vi "Inpaint.vi"(0 "image in":refnum<class "MSC Image.lvclass">, 1 "mask image in":refnum<class "MSC Image.lvclass">, 2 "Radius":i32=5, 3 "Algorithm":T1, 5 "error in (no error)":errorcluster) -> (14 "image out":refnum<class "MSC Image.lvclass">, 15 "mask image out":refnum<class "MSC Image.lvclass">, 19 "error out":errorcluster)   [LabVIEW 2016, in "MSC Image.lvclass"]
doc: "Restores marked image regions through an inpaint algorithm."
uses:
  MSC Image.lvclass
  Dependencies/x86/MSC I Process32.dll
  controls/Inpaint Algorithm Method.ctl
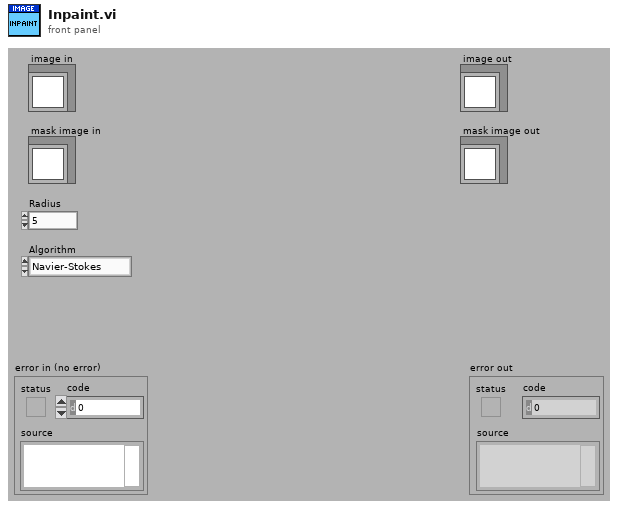
[diagram p1: front panel]
types:
  T1 = typedef "MSC Image.lvclass/Inpaint Algorithm Method.ctl" = enum16{"Navier-Stokes", "Alexandru Telea"}
  T2 = typedef "Image.ctl" = cluster{"Pointer":u64, "Size":T3, "Image Type":T4, "Time Stamp":timestamp, "Variant":variant}
  T3 = typedef "Size.ctl" = cluster{"Cols":i32, "Rows":i32}
  T4 = typedef "Image Type.ctl" = i32
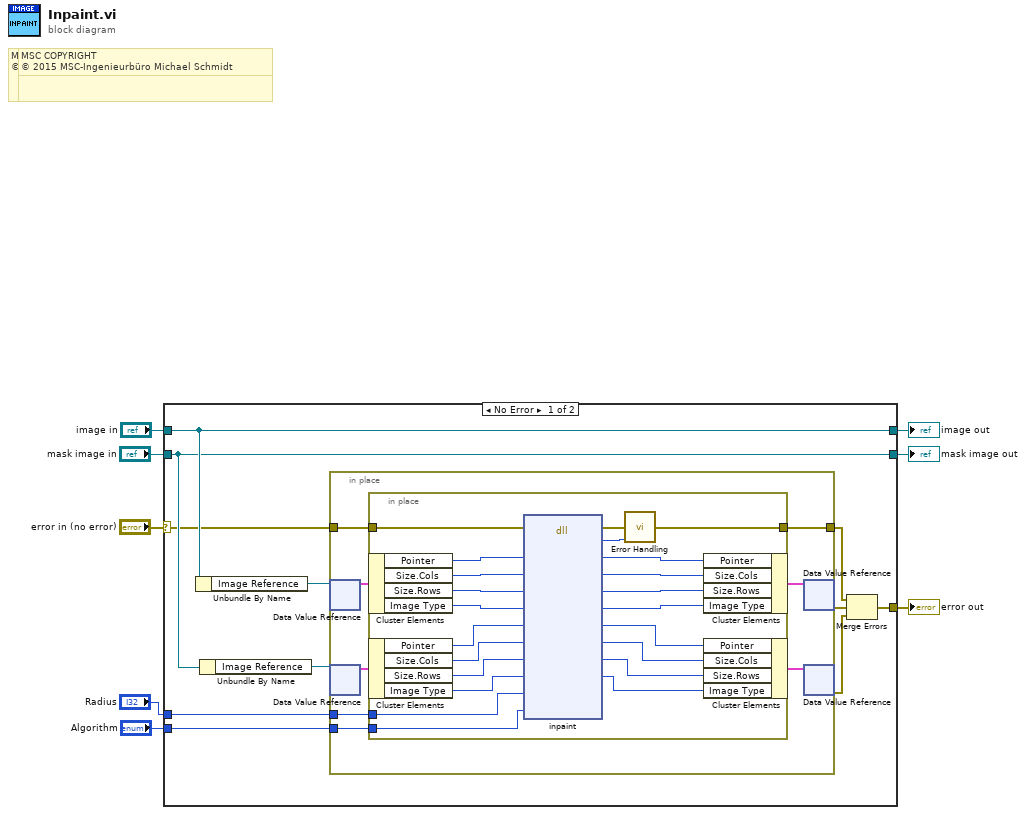
[diagram p0: block diagram]
diagram:
  # "MSC COPYRIGHT\n© 2016 MSC-Ingenieurbüro Michael Schmidt"
  # "MSC COPYRIGHT\n© 2016 MSC-Ingenieurbüro Michael Schmidt"
  # "MSC COPYRIGHT\n© 2015 MSC-Ingenieurbüro Michael Schmidt"
  # "MSC COPYRIGHT\n© 2015 MSC-Ingenieurbüro Michael Schmidt"
  n1 = case shown="No Error" "error in (no error)" {
    selector: "error in (no error)" -> [w9 w52]
    tunnel: [w16 w52] -> w1
    tunnel: [w10 w50] -> w6
    tunnel: "image in" -> [w13 w51]
    tunnel: [w13 w51] -> w7
    tunnel: "mask image in" -> [w10 w50]
    tunnel: "Radius" -> [w15 _]
    tunnel: "Algorithm" -> [w14 _]
    frame No Error {
      n2 = Unbundle By Name(w13) -> ("Image Reference"=w12:refnum<data-value>)
      n3 = Unbundle By Name(w10) -> ("Image Reference"=w11:refnum<data-value>)
      n4 = in-place {
        in-place-border: w9 -> [w25]
        in-place-border: [w24] -> w19
        in-place-border: w15 -> [w21]
        in-place-border: w14 -> [w20]
        n5 = in-place-dvr #1(w12) -> (w26:T2)  [unwired: 1 out]
        n6 = in-place-dvr #2(w11) -> (w23:T2)  [unwired: 1 out]
        n7 = in-place {
          in-place-border: w25 -> [w30]
          in-place-border: [w49] -> w24
          in-place-border: w21 -> [w29]
          in-place-border: w20 -> [w28]
          n8 = in-place-cluster #3(w26) -> ("Pointer"=w48:u64, "Size.Cols"=w47:i32, "Size.Rows"=w46:i32, "Image Type"=w45:T4)
          n9 = in-place-cluster #4(w23) -> ("Pointer"=w44:u64, "Size.Cols"=w43:i32, "Size.Rows"=w42:i32, "Image Type"=w41:T4)
          n10 = dll-call lib="C:/Users/MSC/LabVIEW Projekte/LV 2014/MSC I-Process/user.lib/MSC-I Process/Dependencies/x86/MSC I Process*.dll" fn="inpaint"(error in=w30, "pointer"=w48, "cols"=w47, "rows"=w46, "type"=w45, "pointerMask"=w44, "colsMask"=w43, "rowsMask"=w42, "typeMask"=w41, "radius"=w29, "flag"=w28) -> (error out=w31:errorcluster, "error"=w32:i32, "pointer"=w36:u64, "cols"=w35:i32, "rows"=w34:i32, "type"=w33:i32, "pointerMask"=w40:u64, "colsMask"=w39:i32, "rowsMask"=w38:i32, "typeMask"=w37:i32)  [unwired: 4 in, 1 out]
          n11 = call "Error Handling.vi"("error in (no error)"=w31, "return type"=w32) -> ("error out"=w49:errorcluster)  [unwired: 12 in, 1 out]
          n12 = in-place-cluster #3("Pointer"=w36, "Size.Cols"=w35, "Size.Rows"=w34, "Image Type"=w33) -> (w27:T2)
          n13 = in-place-cluster #4("Pointer"=w40, "Size.Cols"=w39, "Size.Rows"=w38, "Image Type"=w37) -> (w22:T2)
        }
        n14 = in-place-dvr #1(w27) -> (w18:errorcluster)  [unwired: 1 out]
        n15 = in-place-dvr #2(w22) -> (w17:errorcluster)  [unwired: 1 out]
      }
      n16 = Merge Errors(w19, w18, w17) -> (w16:errorcluster)
    }
    frame Error {
    }
  }
  "error out" <- w1
  "image out" <- w7
  "mask image out" <- w6
